vi "Klinger CheckOptions.vi"(0 "Message Cont":string caption="Message de statut", 3 "error in":errorcluster) -> (7 "Statut":bool, 10 "error out":errorcluster)   [LabVIEW 2010]
doc: "Ce VI vérifie si toutes les options de statut sont activée"
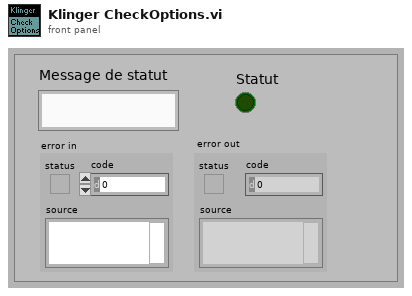
[diagram p1: front panel]
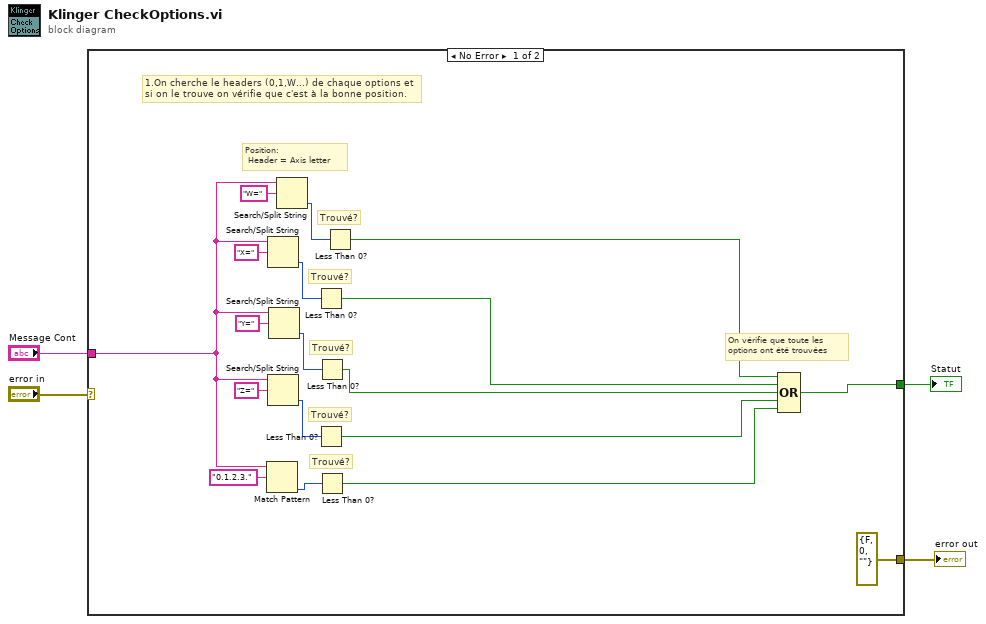
[diagram p0: block diagram]
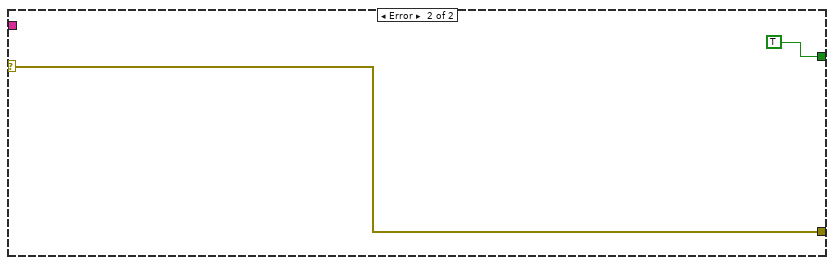
[diagram p2: hidden frame]
diagram:
  n1 = case shown="No Error" "error in" {
    selector: "error in" -> [_ w23]
    tunnel: [errorcluster {"status"=FALSE, "code"=0, "source"=""} ("error IO") w23] -> w4
    tunnel: [w21 TRUE ("Statut")] -> w3
    tunnel: "Message Cont" -> [w8 _]
    frame No Error {
      # "Trouvé?"
      # "Trouvé?"
      # "Trouvé?"
      # "Trouvé?"
      # "1.On cherche le headers (0,1,W...) de chaque options et\nsi on le trouve on vérifie que c'est à la bonne position."
      # "Trouvé?"
      # "On vérifie que toute les \noptions ont été trouvées"
      # "Position:\n Header = Axis letter"
      n2 = Match Pattern(string=w8, regular expression="0.1.2.3.") -> (offset past match=w6:i32)  [unwired: 1 in, 3 out]
      n3 = Search/Split String(string=w8, search string/char (-)="X=") -> (offset of match=w16:i32)  [unwired: 1 in, 2 out]
      n4 = Search/Split String(string=w8, search string/char (-)="Z=") -> (offset of match=w12:i32)  [unwired: 1 in, 2 out]
      n5 = Search/Split String(string=w8, search string/char (-)="Y=") -> (offset of match=w15:i32)  [unwired: 1 in, 2 out]
      n6 = Search/Split String(string=w8, search string/char (-)="W=") -> (offset of match=w22:i32)  [unwired: 1 in, 2 out]
      n7 = Less Than 0?(x=w16) -> (x < 0?=w11:bool)
      n8 = Less Than 0?(x=w12) -> (x < 0?=w9:bool)
      n9 = Less Than 0?(x=w15) -> (x < 0?=w10:bool)
      n10 = Less Than 0?(x=w6) -> (x < 0?=w5:bool)
      n11 = Less Than 0?(x=w22) -> (x < 0?=w19:bool)
      n12 = Compound Arithmetic op=OR(w19, w11, w10, w9, w5) -> (w21:bool)
    }
    frame Error {
    }
  }
  "error out" <- w4
  "Statut" <- w3
